vi "Record Trace.vi"(8 "error in (no error)":errorcluster, 10 "Trace":refnum<class "Trace.lvclass">, 11 "System Actor in":refnum<class "System Actor.lvclass">) -> (0 "error out":errorcluster, 3 "System Actor out":refnum<class "System Actor.lvclass">)   [LabVIEW 2014, in "Robot Actor Framework.lvlib" / "System Actor.lvlib" / "System Actor.lvclass"]
uses:
  System Actor.lvclass
  Trace/Trace Class/Trace.lvclass
  Utilities/Utilities.lvlib
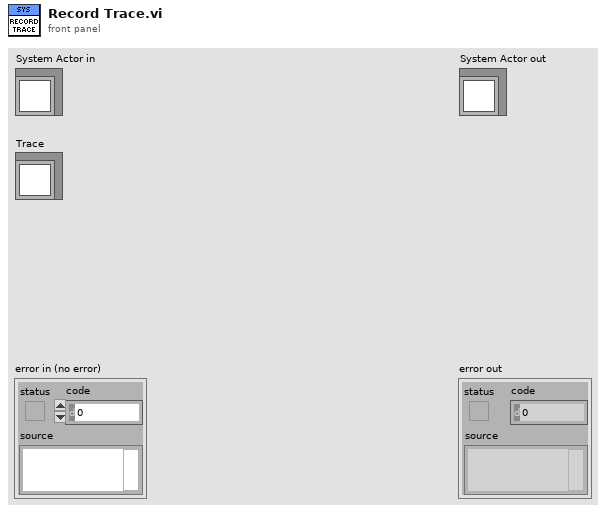
[diagram p1: front panel]
types:
  T1 = enum16{"Critical", "Error", "Warning", "Informational", "Debug"}
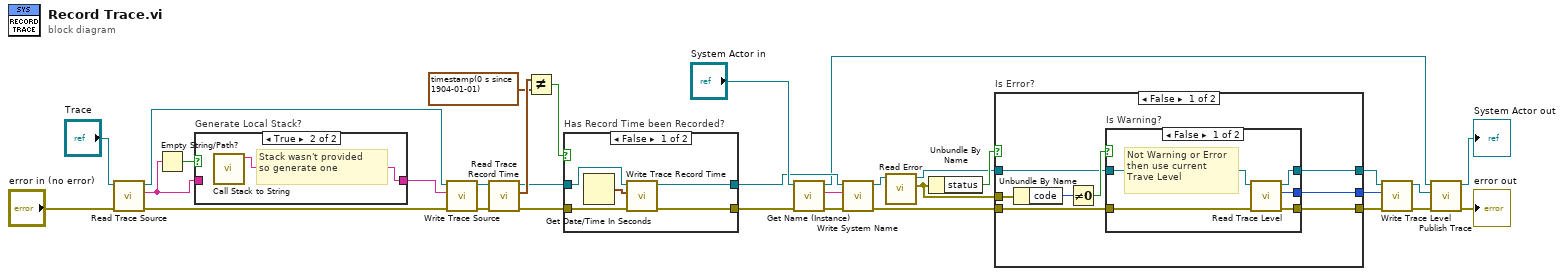
[diagram p0: block diagram]
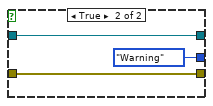
[diagram p3: hidden frame]
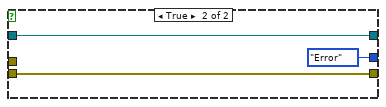
[diagram p4: hidden frame]
diagram:
  n1 = call-dynamic "Read Trace Source.vi"("error in (no error)"="error in (no error)", "Trace in"="Trace") -> ("error out"=w10:errorcluster, "Trace Source"=w26:string, "Trace out"=w13:refnum<class "Trace.lvclass">)  [unwired: 7 in]
  n2 = Empty String/Path?(string/path=w26) -> (empty?=w30:bool)
  n3 = case "Generate Local Stack?" shown="True" w30 {
    tunnel: w26 -> [w33 _]
    tunnel: [w33 w34] -> w12
    frame False {
    }
    frame True {
      # "Stack wasn't provided\nso generate one"
      n4 = call "Call Stack to String.vi"() -> ("Call Stack String"=w34:string)  [unwired: 11 in]
    }
  }
  n5 = call-dynamic "Write Trace Source.vi"("error in (no error)"=w10, "Trace Source"=w12, "Trace in"=w13) -> ("error out"=w9:errorcluster, "Trace out"=w11:refnum<class "Trace.lvclass">)  [unwired: 7 in]
  n6 = call-dynamic "Read Trace Record Time.vi"("error in (no error)"=w9, "Trace in"=w11) -> ("error out"=w15:errorcluster, "Trace Record Time"=w21:timestamp, "Trace out"=w18:refnum<class "Trace.lvclass">)  [unwired: 7 in]
  n7 = Not Equal?(x=w21, y=timestamp(0 s since 1904-01-01)) -> (x != y?=w19:bool)
  n8 = case "Has Record Time been Recorded?" shown="False" w19 {
    tunnel: w18 -> [w39 w41]
    tunnel: [w38 w41] -> w17
    tunnel: w15 -> [w36 w40]
    tunnel: [w35 w40] -> w14
    frame False {
      n9 = Get Date/Time In Seconds() -> (seconds since 1Jan1904=w37:timestamp)
      n10 = call-dynamic "Write Trace Record Time.vi"("error in (no error)"=w36, "Trace Record Time"=w37, "Trace in"=w39) -> ("error out"=w35:errorcluster, "Trace out"=w38:refnum<class "Trace.lvclass">)  [unwired: 7 in]
    }
    frame True {
    }
  }
  n11 = call-dynamic "Get Name (Instance).vi"("error in (no error)"=w14, "System Actor in"="System Actor in") -> ("error out"=w23:errorcluster, "System Name - Instance"=w22:string, "System Actor out"=w8:refnum<class "System Actor.lvclass">)  [unwired: 7 in]
  n12 = call-dynamic "Write System Name.vi"("error in (no error)"=w23, "System Name (Inst)"=w22, "Trace in"=w17) -> ("error out"=w7:errorcluster, "Trace out"=w4:refnum<class "Trace.lvclass">)  [unwired: 7 in]
  n13 = call-dynamic "Read Error.vi"("Trace in"=w4) -> ("Error"=w1:errorcluster, "Trace out"=w3:refnum<class "Trace.lvclass">)  [unwired: 8 in, 1 out]
  n14 = Unbundle By Name(w1) -> ("status"=w28:bool)
  n15 = case "Is Error?" shown="False" w28 {
    tunnel: w1 -> [w49 _]
    tunnel: [w46 T1."Error" ("Trace Level")] -> w27
    tunnel: w3 -> [w45 w59]
    tunnel: [w44 w59] -> w16
    tunnel: w7 -> [w43 w58]
    tunnel: [w42 w58] -> w6
    frame False {
      n16 = Unbundle By Name(w49) -> ("code"=w48:i32)
      n17 = Not Equal To 0?(x=w48) -> (x != 0?=w47:bool)
      n18 = case "Is Warning?" shown="False" w47 {
        tunnel: [w54 T1."Warning" ("Trace Level")] -> w46
        tunnel: w45 -> [w53 w56]
        tunnel: [w52 w56] -> w44
        tunnel: w43 -> [w51 w55]
        tunnel: [w50 w55] -> w42
        frame False {
          # "Not Warning or Error\nthen use current\nTrave Level"
          n19 = call-dynamic "Read Trace Level.vi"("error in (no error)"=w51, "Trace in"=w53) -> ("error out"=w50:errorcluster, "Trace Level"=w54:T1, "Trace out"=w52:refnum<class "Trace.lvclass">)  [unwired: 7 in]
        }
        frame True {
        }
      }
    }
    frame True {
    }
  }
  n20 = call-dynamic "Write Trace Level.vi"("error in (no error)"=w6, "Trace Level"=w27, "Trace in"=w16) -> ("error out"=w25:errorcluster, "Trace out"=w29:refnum<class "Trace.lvclass">)  [unwired: 7 in]
  n21 = call-dynamic "Publish Trace.vi"("error in (no error)"=w25, "Trace In"=w29, "System Actor in"=w8) -> ("error out"=→"error out":errorcluster, "System Actor out"=→"System Actor out":refnum<class "System Actor.lvclass">)  [unwired: 7 in]
